vi "Configure Probe External.vi"(7 "External Coupling Adapter (0: None)":i32(ring) items=["None", "AC"], 8 "error in (no error)":errorcluster, 9 "External Adapter (0: None)":i32(ring) items=["None", "Divide by 10", "Divide by 20", "Divide by 100"], 10 "Channel (1: Channel 1)":i32(ring)=1 items=["Channel 1"=1, "Channel 2"=2, "Channel 3"=3, "Channel 4"=4], 11 "VISA resource name":refnum<visa-resource-name>) -> (0 "error out":errorcluster, 3 "VISA resource name out":refnum<visa-resource-name>)   [LabVIEW 2020, in "Agilent 90000 Series.lvlib"]
doc: "Configures probe external adapter control and external coupling adapter control.\n\n<B>Note:</B>\nThis VI is valid only for the 1153A, 1154A, and 1159A probes."
uses:
  Agilent 90000 Series.lvlib
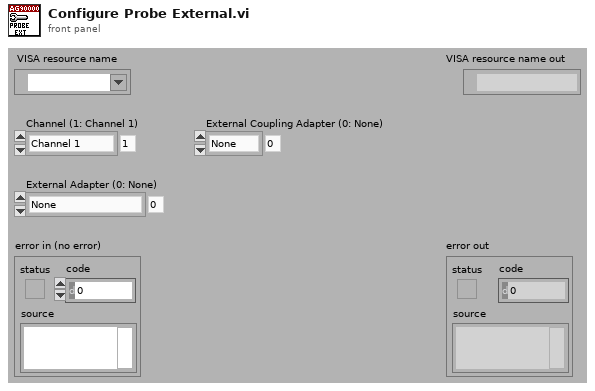
[diagram p1: front panel]
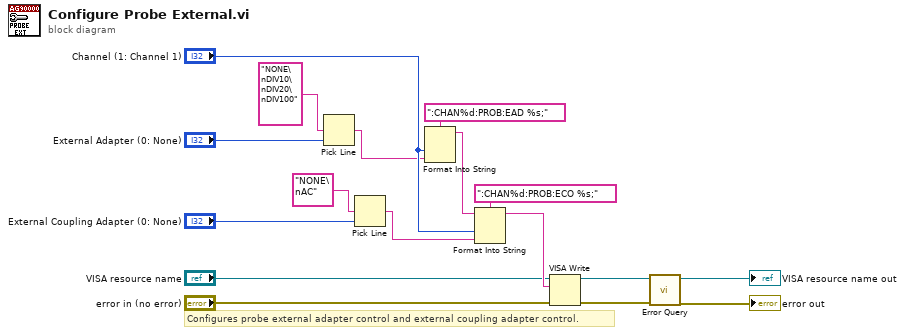
[diagram p0: block diagram]
diagram:
  # "Configures probe external adapter control and external coupling adapter control."
  n1 = Pick Line(multi-line string="NONE\nDIV10\nDIV20\nDIV100", line index="External Adapter (0: None)") -> (output string=w13:string)  [unwired: 1 out]
  n2 = Pick Line(multi-line string="NONE\nAC", line index="External Coupling Adapter (0: None)") -> (output string=w8:string)  [unwired: 1 out]
  n3 = Format Into String(format string=":CHAN%d:PROB:EAD %s;", "Channel (1: Channel 1)", w13) -> (resulting string=w10:string)  [unwired: 2 in, 1 out]
  n4 = Format Into String(format string=":CHAN%d:PROB:ECO %s;", initial string=w10, "Channel (1: Channel 1)", w8) -> (resulting string=w7:string)  [unwired: 1 in, 1 out]
  n5 = VISA Write(VISA resource name="VISA resource name", write buffer=w7, error in (no error)="error in (no error)") -> (VISA resource name out=w4:refnum<visa-resource-name>, error out=w3:errorcluster)  [unwired: 1 out]
  n6 = call "Error Query.vi"("error in (no error)"=w3, "VISA resource name"=w4) -> ("error out"=→"error out":errorcluster, "VISA resource name out"=→"VISA resource name out":refnum<visa-resource-name>)  [unwired: 8 out]
